vi "CCC Client Read.vi"(8 "error in (no error)":errorcluster, 11 "CCC Connection ID in":T1) -> (0 "error out":errorcluster, 3 "CCC Connection ID out":T1)   [LabVIEW 2010]
doc: "This VI is used by the client side of the CVT Client Communication API to read CVT values from the server."
uses:
  ccc_ConnectionID.ctl
  <vilib>/NI/STM/compatibility/stm_TCP Connection Info.ctl
  <vilib>/NI/STM/compatibility/stm_MetaDataElement.ctl
  ccc_TagConfiguration.ctl
  <vilib>/NI/Current Value Table/Compatibility/_SubVIs/TypeDefs/cvt_Data Types.ctl
  ccc_TagDirection.ctl
  ccc_Convert From Compatibility TagConfig.vi
  NI_CCC.lvlib
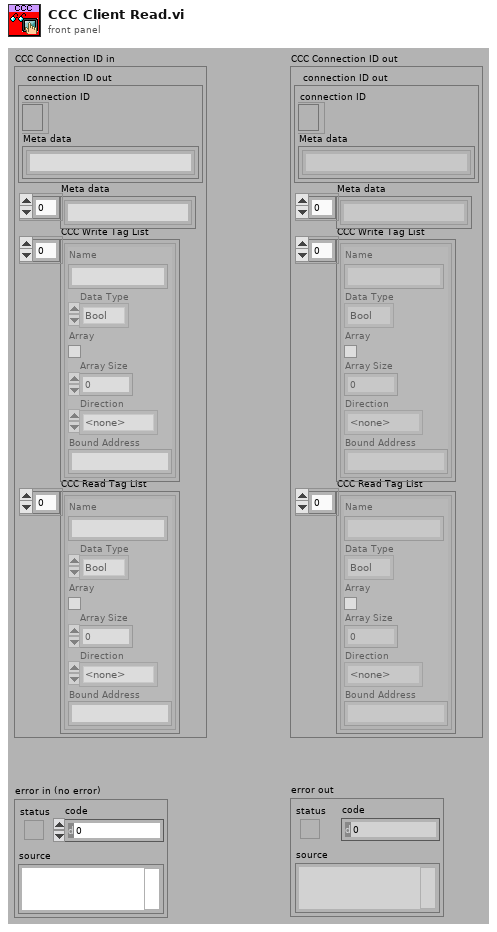
[diagram p1: front panel]
types:
  T1 = typedef "ccc_ConnectionID.ctl" = cluster{"connection ID out":T2, "Meta data":T3[], "CCC Write Tag List":T4[], "CCC Read Tag List":T4[]}
  T2 = typedef "stm_TCP Connection Info.ctl" = cluster{"connection ID":refnum<k5>, "Meta data":T3[]}
  T3 = typedef "stm_MetaDataElement.ctl" = string
  T4 = typedef "ccc_TagConfiguration.ctl" = cluster{"Name":string, "Data Type":T5, "Array":bool, "Array Size":u32, "Direction":T6, "Bound Address":string}
  T5 = typedef "cvt_Data Types.ctl" = enum16{"Bool", "U8", "I32", "Double", "String", "Enum"}
  T6 = typedef "ccc_TagDirection.ctl" = enum32{"<none>", "Read", "Write"}
  T7 = typedef "NI_CCC.lvlib/Connection ID.ctl" = cluster{"connection ID out":T8, "meta data":T9[], "write tag list":T10[], "read tag list":T10[]}
  T8 = typedef "NI STM.lvlib/TCP Connection Info.ctl" = cluster{"connection ID":refnum<k5>, "Meta data":T9[]}
  T9 = typedef "NI STM.lvlib/MetaDataElement.ctl" = string
  T10 = typedef "NI_CCC.lvlib/Tag Configuration.ctl" = cluster{"name":string, "data type":T11, "direction":T12, "bound address":string}
  T11 = typedef "Current Value Table.lvlib/Data Types.ctl" = enum16{"Double", "Single", "I64", "I32", "I16", "I8", "U64", "U32", "U16", "U8", "String", "Boolean"}
  T12 = typedef "NI_CCC.lvlib/Tag Direction.ctl" = enum32{"<none>", "Read", "Write"}
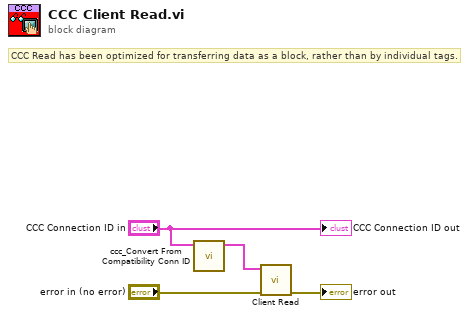
[diagram p0: block diagram]
diagram:
  # "CCC Read has been optimized for transferring data as a block, rather than by individual tags."
  n1 = call "ccc_Convert From Compatibility Conn ID.vi"("old connection ID"="CCC Connection ID in") -> ("new connection ID"=w4:T7)  [unwired: 10 in]
  n2 = call "Client Read.vi"("error in"="error in (no error)", "connection ID in"=w4) -> ("error out"=→"error out":errorcluster)  [unwired: 8 in, 1 out]
  "CCC Connection ID out" <- "CCC Connection ID in"
